vi "EvaluatePoint.vi"(8 "error in (no error)":errorcluster, 9 "Game":refnum<class "Game.lvclass">, 10 "Point":dbl[](array[numeric]), 11 "PrimaryAttackerShot in":refnum<class "PrimaryAttackerShot.lvclass">) -> (0 "error out":errorcluster, 2 "Evaluation":dbl, 3 "PrimaryAttackerShot out":refnum<class "PrimaryAttackerShot.lvclass">)   [LabVIEW 2023, in "PrimaryAttackerShot.lvclass"]
uses:
  PrimaryAttackerShot.lvclass
  Game_class/Game.lvclass
  Evaluator_class/Evaluator.lvclass
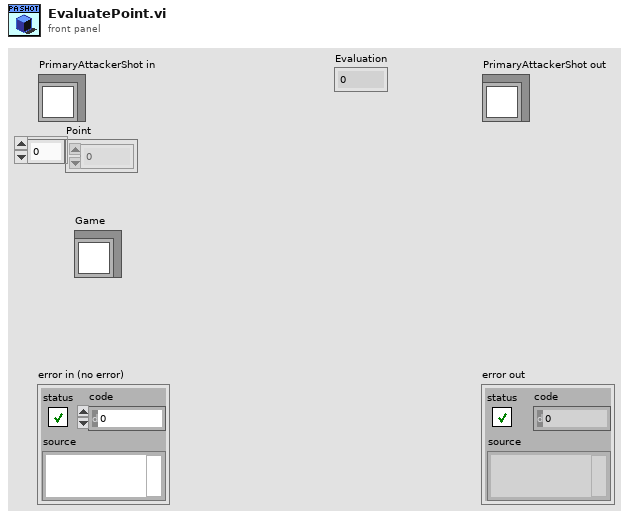
[diagram p1: front panel]
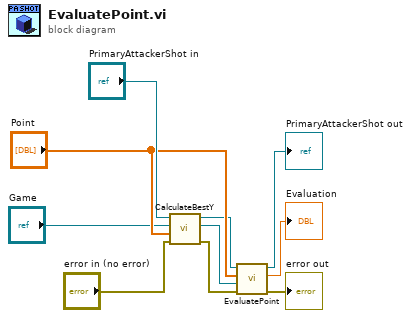
[diagram p0: block diagram]
diagram:
  n1 = call-dynamic "CalculateBestY.vi"("error in (no error)"="error in (no error)", "Point"="Point", "Game"="Game", "Evaluator in"="PrimaryAttackerShot in") -> ("error out"=w3:errorcluster, "Game out"=w2:refnum<class "Game.lvclass">, "Evaluator out"=w1:refnum<class "PrimaryAttackerShot.lvclass">)  [unwired: 5 in]
  n2 = call-parent "EvaluatePoint.vi"("error in (no error)"=w3, "Game"=w2, "Point"="Point", "Evaluator in"=w1) -> ("error out"=→"error out":errorcluster, "Evaluation"=→"Evaluation":dbl, "Evaluator out"=→"PrimaryAttackerShot out":refnum<class "PrimaryAttackerShot.lvclass">)  [unwired: 5 in]
